vi "画面亮度调节.vi"() -> ()   [LabVIEW 2020]
uses:
  <vilib>/userdefined/High Color/IMAQdx.ctl
  <vilib>/vision/driver/NI_Vision_Acquisition_Software.lvlib
  <vilib>/vision/NI_Vision_Development_Module.lvlib
panel:
  in  "停止":bool
  out "Image":T1(plugin-control)
  in  "枚举":enum16{"ALL", "R", "G", "B"}(ring)
  in  "Gamma":sgl(slide) scale=0.0..2.0
  in  "Contrast":sgl(slide) scale=0.0..90.0
  in  "Brightness":sgl(slide) scale=0.0..256.0
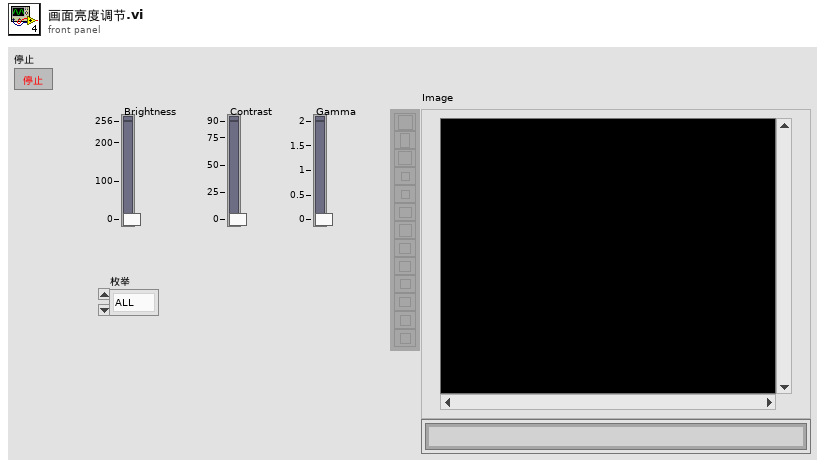
[diagram p1: front panel]
types:
  T1 = typedef "IMAQ Image.ctl" = refnum<image>
  T2 = cluster{"Brightness":sgl, "Contrast":sgl, "Gamma":sgl}
  T3 = typedef "IMAQdx.ctl" = refnum<k21>
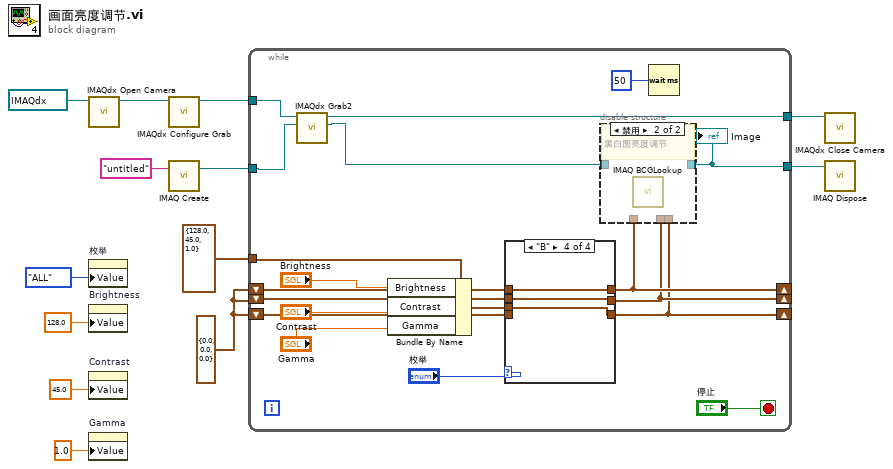
[diagram p0: block diagram]
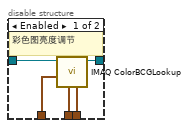
[diagram p2: hidden frame]
diagram:
  w1 = T2 {"Brightness"=0.0, "Contrast"=0.0, "Gamma"=0.0} ("Red BCG Values")
  n1 = call <vilib>:"IMAQdx Open Camera.vi"("Session In"=T3 "cam1") -> ("Session Out"=w12:T3)  [unwired: 9 in, 1 out]
  n2 = property on="枚举" class="Enum (严格)"("Value"=enum16{"ALL", "R", "G", "B"}."ALL" ("枚举")) -> ()  [unwired: 2 in, 2 out]
  n3 = property on="Brightness" class="Slide (严格)"("Value"=sgl 128.0 ("Brightness")) -> ()  [unwired: 2 in, 2 out]
  n4 = property on="Contrast" class="Slide (严格)"("Value"=sgl 45.0 ("Contrast")) -> ()  [unwired: 2 in, 2 out]
  n5 = property on="Gamma" class="Slide (严格)"("Value"=sgl 1.0 ("Gamma")) -> ()  [unwired: 2 in, 2 out]
  n6 = call <vilib>:"IMAQdx Configure Grab.vi"("Session In"=w12) -> ("Session Out"=w10:T3)  [unwired: 9 in, 1 out]
  n7 = call "IMAQ Create"("Image Name"="untitled") -> ("New Image"=w9:T1)  [unwired: 4 in, 1 out]
  n8 = while {
    tunnel: w10 -> [w31]
    tunnel: w9 -> [w30]
    tunnel: [w29] -> w2
    tunnel: T2 {"Brightness"=128.0, "Contrast"=45.0, "Gamma"=1.0} ("Red BCG Values") -> [w27]
    tunnel: [w21] -> w3
    shift-right: [w17] -> _
    shift-left: w1 -> [w14]
    shift-right: [w18] -> _
    shift-left: w1 -> [w15]
    shift-right: [w19] -> _
    shift-left: w1 -> [w16]
    stop <- "停止" stop-if-true
    n9 = call <vilib>:"IMAQdx Grab2.vi"("Image In"=w30, "Session In"=w31) -> ("Image Out"=w28:T1, "Session Out"=w29:T3)  [unwired: 6 in, 2 out]
    n10 = Bundle By Name(cluster=w27, "Brightness"="Brightness", "Contrast"="Contrast", "Gamma"="Gamma") -> (w22:T2)
    n11 = case shown="\"B\"" "枚举" {
      tunnel: w22 -> [w38 w41 w44 w47]
      tunnel: [w38 w41 w43 w45] -> w19
      tunnel: [w38 w40 w44 w46] -> w18
      tunnel: [w38 w39 w42 w47] -> w17
      tunnel: w16 -> [_ _ w43 w45]
      tunnel: w15 -> [_ w40 _ w46]
      tunnel: w14 -> [_ w39 w42 _]
      frame "ALL", Default {
      }
      frame "R" {
      }
      frame "G" {
      }
      frame "B" {
      }
    }
    n12 = disable-structure shown="禁用" {
      disable-tunnel: w28 -> [w37 _]
      disable-tunnel: [w36 _] -> w21
      disable-tunnel: w19 -> [w35 _]
      disable-tunnel: w18 -> [w34 _]
      disable-tunnel: w17 -> [w33 _]
      frame Enabled {
        # "彩色图亮度调节"
        n13 = call "IMAQ ColorBCGLookup"("Blue BCG Values"=w33, "Green BCG Values"=w34, "Red BCG Values"=w35, "Image Src"=w37) -> ("Image Dst Out"=w36:T1)  [unwired: 6 in, 1 out]
      }
      frame Disabled {
        # "黑白图亮度调节"
        n14 = call "IMAQ BCGLookup"() -> ()  [unwired: 7 in, 2 out]
      }
    }
    "Image" <- w21
    n15 = Wait (ms)(milliseconds to wait=u32 50 ("等待时间（毫秒）")) -> ()  [unwired: 1 out]
  }
  n16 = call <vilib>:"IMAQdx Close Camera.vi"("Session In"=w2) -> ()  [unwired: 10 in, 1 out]
  n17 = call "IMAQ Dispose"("Image"=w3) -> ()  [unwired: 5 in, 1 out]
